vi "log_record_file.vi"(8 "error in":errorcluster, 11 "st_LogEvent":string) -> (0 "error out":errorcluster)   [LabVIEW 2026]
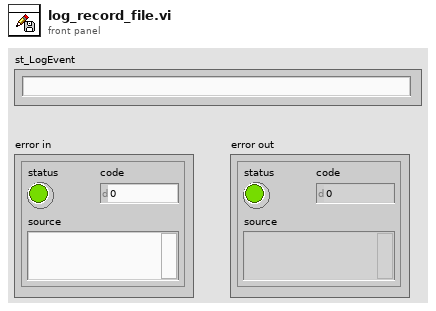
[diagram p1: front panel]
types:
  T1 = enum16{"open", "replace", "create", "open or create", "replace or create", "replace or create with confirmation"}
  T2 = cluster{"second":string, "minute":string, "hour":string, "day":string, "month":string, "year":string}
  T3 = typedef "LVDateTimeRec.ctl" = cluster{"fractional second":dbl, "second":i32, "minute":i32, "hour":i32, "day of month":i32, "month":i32, "year":i32, "day of week":i32, "day of year":i32, "DST":i32}
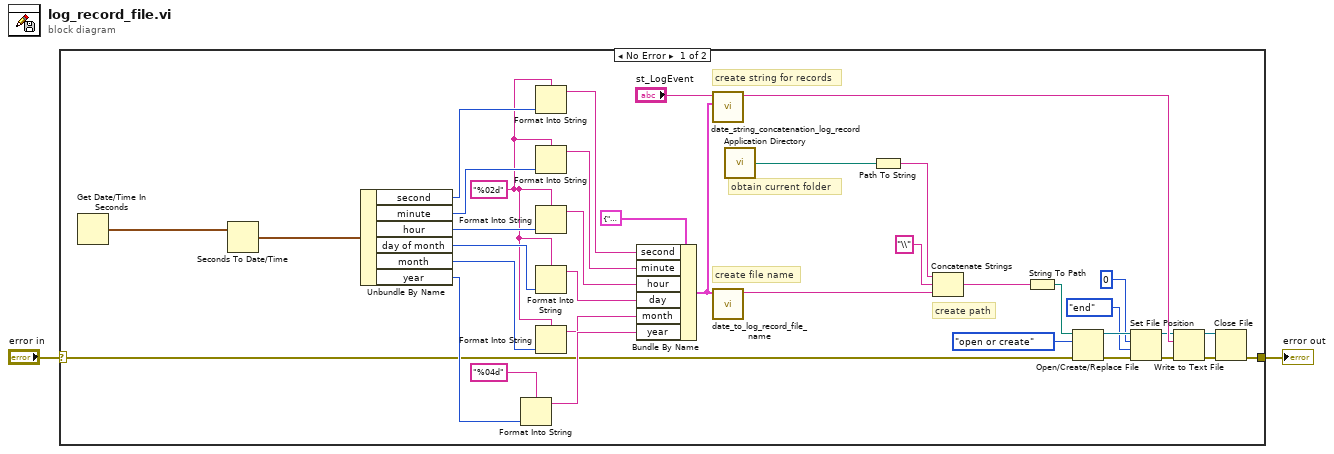
[diagram p0: block diagram]
diagram:
  n1 = case shown="No Error" "error in" {
    selector: "error in" -> [w21 w40]
    tunnel: [w20 w40] -> w1
    frame No Error {
      w10 = "%02d"
      # "create path"
      # "obtain current folder"
      # "create string for records"
      # "create file name"
      n2 = Get Date/Time In Seconds() -> (seconds since 1Jan1904=w38:timestamp)
      n3 = Seconds To Date/Time(time stamp (now)=w38) -> (date time rec=w39:T3)  [unwired: 1 in]
      n4 = Unbundle By Name(w39) -> ("second"=w37:i32, "minute"=w36:i32, "hour"=w35:i32, "day of month"=w34:i32, "month"=w33:i32, "year"=w32:i32)
      n5 = Format Into String(format string="%04d", w32) -> (resulting string=w30:string)  [unwired: 2 in, 1 out]
      n6 = Format Into String(format string=w10, w37) -> (resulting string=w29:string)  [unwired: 2 in, 1 out]
      n7 = Format Into String(format string=w10, w36) -> (resulting string=w28:string)  [unwired: 2 in, 1 out]
      n8 = Format Into String(format string=w10, w35) -> (resulting string=w27:string)  [unwired: 2 in, 1 out]
      n9 = Format Into String(format string=w10, w34) -> (resulting string=w26:string)  [unwired: 2 in, 1 out]
      n10 = Format Into String(format string=w10, w33) -> (resulting string=w25:string)  [unwired: 2 in, 1 out]
      n11 = Bundle By Name(cluster=T2 {"second"="", "minute"="", "hour"="", "day"="", "month"="", "year"=""}, "second"=w29, "minute"=w28, "hour"=w27, "day"=w26, "month"=w25, "year"=w30) -> (w23:T2)
      n12 = call "date_string_concatenation_log_record.vi"("Cluster"=w23, "st_LogEvent"="st_LogEvent") -> ("st_logrecord"=w12:string)  [unwired: 9 in]
      n13 = call "date_to_log_record_file_name.vi"("Cluster"=w23) -> ("st_logfilename"=w15:string)  [unwired: 10 in]
      n14 = call <vilib>:"Application Directory.vi"() -> ("Application Directory"=w18:path)
      n15 = Path To String(path=w18) -> (string=w16:string)
      n16 = Concatenate Strings(w16, "\\", w15) -> (w14:string)
      n17 = String To Path(string=w14) -> (path=w13:path)
      n18 = Open/Create/Replace File(file path (use dialog)=w13, error in=w21, operation (0:open)=T1."open or create") -> (refnum out=w8:refnum<file>, error out=w7:errorcluster)  [unwired: 3 in, 1 out]
      n19 = Set File Position(offset (in bytes) (0)=i64 0, refnum=w8, from (0:start)=enum16{"start", "end", "current"}."end", error in=w7) -> (refnum out=w3:refnum<file>, error out=w6:errorcluster)
      n20 = Write to Text File(file (use dialog)=w3, text=w12, error in=w6) -> (refnum out=w19:refnum<file>, error out=w22:errorcluster)  [unwired: 1 in, 1 out]
      n21 = Close File(refnum=w19, error in=w22) -> (error out=w20:errorcluster)  [unwired: 1 out]
    }
    frame Error {
    }
  }
  "error out" <- w1
